vi "Equation of Motion.vi"(0 "torque":dbl[](array[numeric])=[0.0, 0.0, 0.0], 1 "v10":dbl[](array[numeric])=[-1.0, 0.0, 0.0], 2 "v20":dbl[](array[numeric])=[-1.0, 0.0, 0.0], 3 "v30":dbl[](array[numeric])=[-1.0, 0.0, 0.0], 5 "inertia":dbl[](array[numeric])=[0.0, 0.0, 0.0], 7 "damping":dbl[](array[numeric])=[0.0, 0.0, 0.0], 9 "R":T1, 11 "omega":dbl[](array[numeric]), 12 "dt":dbl=0.001) -> (4 "v1d":dbl[](array[numeric]) format="%.2f", 6 "v2d":dbl[](array[numeric]) format="%.2f", 8 "v3d":dbl[](array[numeric]) format="%.2f", 10 "R'":T1, 15 "omega'":dbl[](array[numeric]))   [LabVIEW 2017]
uses:
  <vilib>/Analysis/Matrix/Datatypes/RealMatrix.ctl
  <vilib>/Analysis/baseanly.llb/Real A x B.vi
  <vilib>/Analysis/baseanly.llb/A x Vector.vi
  <vilib>/Analysis/_algsub.llb/Vector Norm.vi
  <vilib>/Analysis/_algsub.llb/Real Vector Norm.vi
  <vilib>/Analysis/baseanly.llb/Outer Product.vi
  <vilib>/Analysis/baseanly.llb/Real Outer Product.vi
  <vilib>/robotics/Kinematics/Create Lie Group Matrix.vi
  <vilib>/Analysis/7linalg.llb/Create Special Matrix.vi
  <vilib>/Analysis/7linalg.llb/Create Special Real Matrix.vi
  <vilib>/Analysis/Matrix/Numeric/Multiply/Multiply.vi
  <vilib>/Analysis/Matrix/Numeric/Multiply/Multiply - RM,R.vi
  <vilib>/Analysis/Matrix/Numeric/Multiply/Multiply - R,RM.vi
  <vilib>/Analysis/Matrix/Numeric/Add/Add.vi
  <vilib>/Analysis/Matrix/Numeric/Add/Add - RM,RM.vi
  <vilib>/robotics/Kinematics/NI_Kinematics.lvlib
  <vilib>/Analysis/NI_AALBase.lvlib
  <vilib>/Analysis/Matrix/NI_Matrix.lvlib
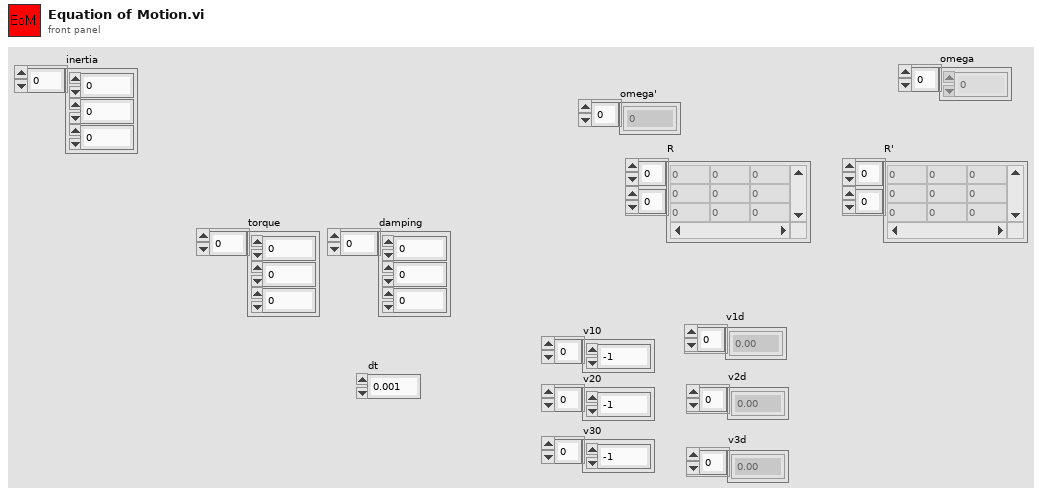
[diagram p1: front panel]
types:
  T1 = typedef "NI_Matrix.lvlib/RealMatrix.ctl" = dbl[][]
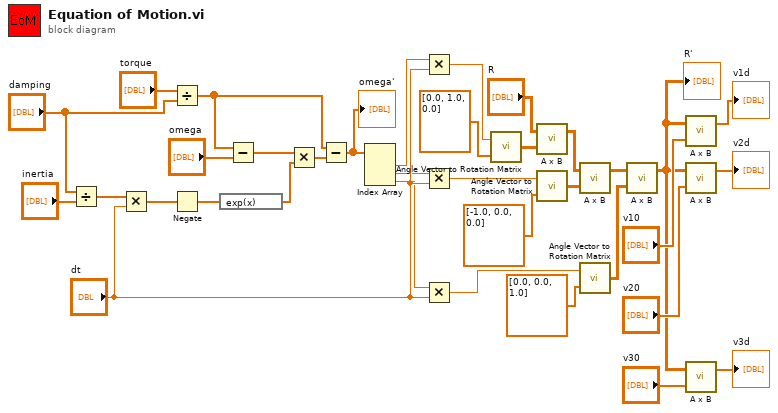
[diagram p0: block diagram]
diagram:
  n1 = Divide(x="damping", y="inertia") -> (x/y=w12:dbl[])
  n2 = Multiply(x=w12, y="dt") -> (x*y=w10:dbl[])
  n3 = Divide(x="torque", y="damping") -> (x/y=w6:dbl[])
  n4 = Negate(x=w10) -> (-x=w9:dbl[])
  n5 = expression code="exp(x)"(w9) -> (w7:dbl[])
  n6 = Subtract(x=w6, y="omega") -> (x-y=w8:dbl[])
  n7 = Multiply(x=w8, y=w7) -> (x*y=w5:dbl[])
  n8 = Subtract(x=w6, y=w5) -> (x-y=w4:dbl[])
  "omega'" <- w4
  n9 = Index Array(array=w4) -> (element #1=w2:dbl, element #2=w1:dbl, element #3=w3:dbl)  [unwired: 3 in]
  n10 = Multiply(x=w2, y="dt") -> (x*y=w34:dbl)
  n11 = Multiply(x=w1, y="dt") -> (x*y=w33:dbl)
  n12 = Multiply(x=w3, y="dt") -> (x*y=w32:dbl)
  n13 = call <vilib>:"Angle Vector to Rotation Matrix.vi"("vector"=dbl[] [0.0, 1.0, 0.0], "angle"=w34) -> ("rotation matrix"=w27:T1)
  n14 = call-poly <vilib>:"A x B.vi"("B"=w27, "A"="R") -> ("A x B"=w26:T1)  [unwired: 1 out]
  n15 = call <vilib>:"Angle Vector to Rotation Matrix.vi"("vector"=dbl[] [-1.0, 0.0, 0.0], "angle"=w33) -> ("rotation matrix"=w25:T1)
  n16 = call-poly <vilib>:"A x B.vi"("B"=w25, "A"=w26) -> ("A x B"=w24:T1)  [unwired: 1 out]
  n17 = call <vilib>:"Angle Vector to Rotation Matrix.vi"("vector"=dbl[] [0.0, 0.0, 1.0], "angle"=w32) -> ("rotation matrix"=w23:T1)
  n18 = call-poly <vilib>:"A x B.vi"("B"=w23, "A"=w24) -> ("A x B"=w20:T1)  [unwired: 1 out]
  "R'" <- w20
  n19 = call-poly <vilib>:"A x B.vi"("Vector"="v10", "A"=w20) -> ("A x Vector"=→"v1d":dbl[])  [unwired: 1 out]
  n20 = call-poly <vilib>:"A x B.vi"("Vector"="v20", "A"=w20) -> ("A x Vector"=→"v2d":dbl[])  [unwired: 1 out]
  n21 = call-poly <vilib>:"A x B.vi"("Vector"="v30", "A"=w20) -> ("A x Vector"=→"v3d":dbl[])  [unwired: 1 out]
